vi "WFM MNGR Create ET Waveform Name.vi"(6 "error in (no error)":errorcluster, 7 "Vmax":dbl, 8 "Vmin":dbl, 9 "Name":string) -> (0 "error out":errorcluster, 2 "result string":string)   [LabVIEW 2016, in "QPA MSMT Waveform Manager.lvclass"]
uses:
  QPA MSMT Waveform Manager.lvclass
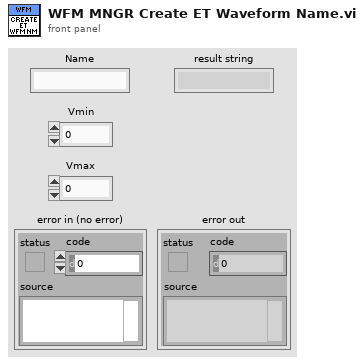
[diagram p1: front panel]
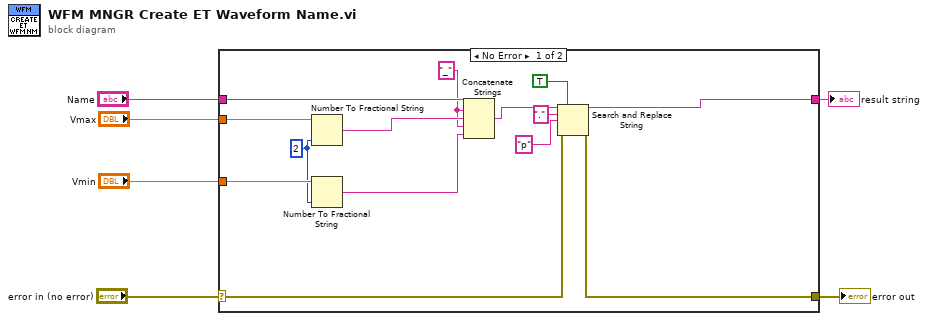
[diagram p0: block diagram]
diagram:
  n1 = case shown="No Error" "error in (no error)" {
    selector: "error in (no error)" -> [w12 w22]
    tunnel: [w11 w22] -> w5
    tunnel: "Name" -> [w17 w21]
    tunnel: "Vmax" -> [w20 _]
    tunnel: "Vmin" -> [w19 _]
    tunnel: [w7 w21] -> w1
    frame No Error {
      w14 = "_" ("string")
      w18 = i16 2 ("precision (6)")
      n2 = Number To Fractional String(number=w20, precision (6)=w18) -> (F-format string=w16:string)  [unwired: 2 in]
      n3 = Number To Fractional String(number=w19, precision (6)=w18) -> (F-format string=w15:string)  [unwired: 2 in]
      n4 = Concatenate Strings(w17, w14, w16, w14, w15) -> (w13:string)
      n5 = Search and Replace String(replace all?=TRUE ("replace all? (F)"), input string=w13, search string=".", replace string="p" ("replace string (\"\")"), error in=w12) -> (result string=w7:string, error out=w11:errorcluster)  [unwired: 3 in, 2 out]
    }
    frame Error {
    }
  }
  "error out" <- w5
  "result string" <- w1
